vi "Get cif_pluginloader_DiscoverResponse.vi"(8 "error in (no error)":errorcluster, 11 "gRPCid":T1) -> (0 "error out":errorcluster, 2 "package_templatemessage":T2, 3 "gRPCid out":T1)   [LabVIEW 2021, in "CIF_PluginLoader_server.lvlib"]
uses:
  CIF_PluginLoader_server.lvlib
  cif_pluginloader_DiscoverResponse.ctl
  cif_pluginloader_DiscoveredPlugin.ctl
  cif_common_Version.ctl
  cif_management_common_PluginMetadata.ctl
  cif_common_Status.ctl
  <vilib>/gRPC/LabVIEW gRPC Library/Shared/grpcId.ctl
  cif_pluginloader_DiscoverResponse_Flat.ctl
  cif_pluginloader_DiscoveredPlugin_Flat.ctl
  cif_common_Version_Flat.ctl
  cif_management_common_PluginMetadata_Flat.ctl
  cif_common_Status_Flat.ctl
  2ed25e12-861d-4677-8ead-ace2906b2041.vi
  <vilib>/gRPC/LabVIEW gRPC Library/Shared/TranslateGrpcError.vi
  FlatToRichcif_pluginloader_DiscoveredPlugin.vi
  FlatToRichcif_common_Status.vi
  FlatToRichcif_common_Version.vi
  FlatToRichcif_management_common_PluginMetadata.vi
  <vilib>/gRPC/LabVIEW gRPC Library/Server API/Server/Get Server DLL Path.vi
  <vilib>/Utility/error.llb/Error Cluster From Error Code.vi
  <vilib>/gRPC/LabVIEW gRPC Library/grpc-lvsupport-release.lvlib
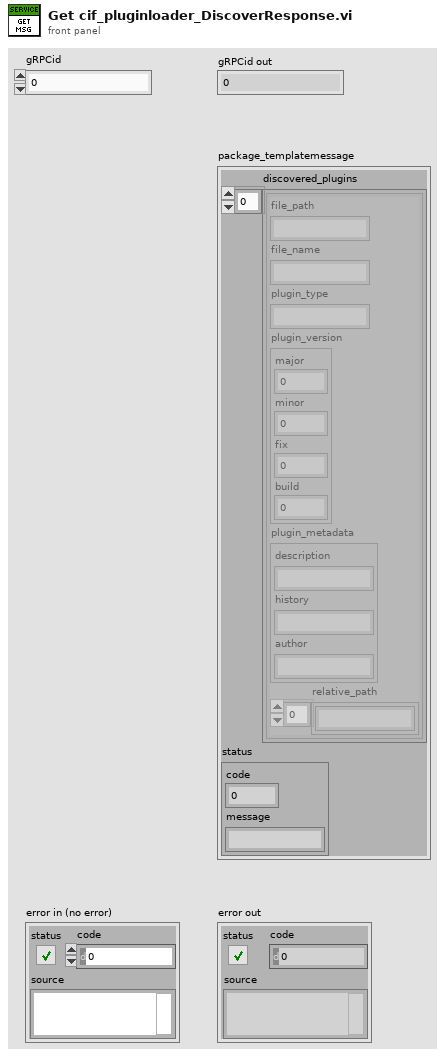
[diagram p1: front panel]
types:
  T1 = typedef "grpc-lvsupport-release.lvlib/grpcId.ctl" = u64
  T2 = typedef "CIF_PluginLoader_server.lvlib/cif_pluginloader_DiscoverResponse.ctl" = cluster{"discovered_plugins":T3[], "status":T6}
  T3 = typedef "CIF_PluginLoader_server.lvlib/cif_pluginloader_DiscoveredPlugin.ctl" = cluster{"file_path":string, "file_name":string, "plugin_type":string, "plugin_version":T4, "plugin_metadata":T5, "relative_path":string[]}
  T4 = typedef "CIF_PluginLoader_server.lvlib/cif_common_Version.ctl" = cluster{"major":u32, "minor":u32, "fix":u32, "build":u32}
  T5 = typedef "CIF_PluginLoader_server.lvlib/cif_management_common_PluginMetadata.ctl" = cluster{"description":string, "history":string, "author":string}
  T6 = typedef "CIF_PluginLoader_server.lvlib/cif_common_Status.ctl" = cluster{"code":i32, "message":string}
  T7 = typedef "CIF_PluginLoader_server.lvlib/cif_pluginloader_DiscoverResponse_Flat.ctl" = cluster{"discovered_plugins":T8[], "status":T11}
  T8 = typedef "CIF_PluginLoader_server.lvlib/cif_pluginloader_DiscoveredPlugin_Flat.ctl" = cluster{"file_path":string, "file_name":string, "plugin_type":string, "plugin_version":T9, "plugin_metadata":T10, "relative_path":string[]}
  T9 = typedef "CIF_PluginLoader_server.lvlib/cif_common_Version_Flat.ctl" = cluster{"major":u32, "minor":u32, "fix":u32, "build":u32}
  T10 = typedef "CIF_PluginLoader_server.lvlib/cif_management_common_PluginMetadata_Flat.ctl" = cluster{"description":string, "history":string, "author":string}
  T11 = typedef "CIF_PluginLoader_server.lvlib/cif_common_Status_Flat.ctl" = cluster{"code":i32, "message":string}
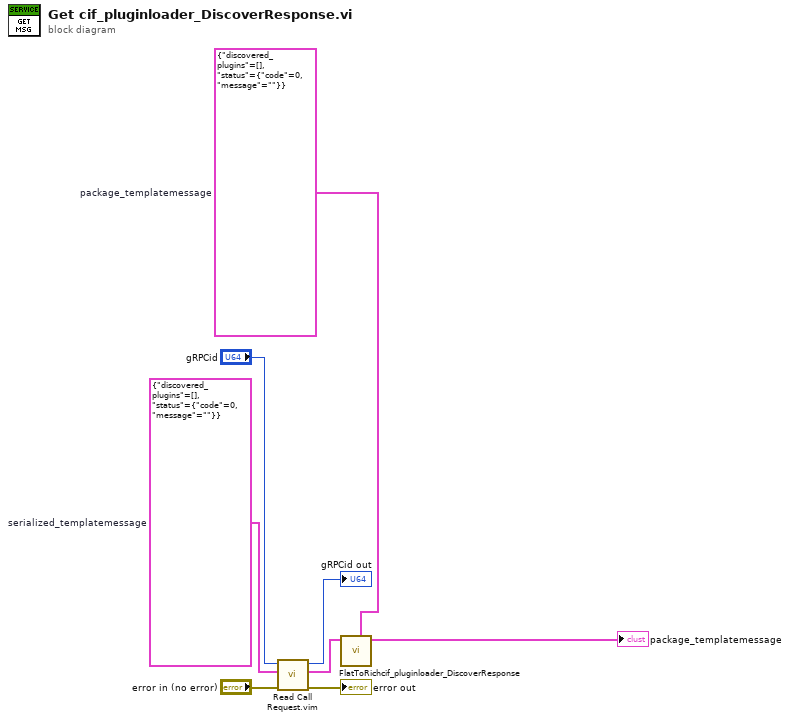
[diagram p0: block diagram]
diagram:
  w6 = T7 {"discovered_plugins"=[], "status"={"code"=0, "message"=""}}  # serialized_templatemessage
  w5 = T2 {"discovered_plugins"=[], "status"={"code"=0, "message"=""}}  # package_templatemessage
  n1 = call "Read Call Request.vim"("error in"="error in (no error)", "Request Type"=w6, "gRPCid in"="gRPCid") -> ("error out"=→"error out":errorcluster, "Request Data"=w4:T7, "gRPCid out"=→"gRPCid out":T1)  [unwired: 6 in]
  n2 = call "FlatToRichcif_pluginloader_DiscoverResponse.vi"("OutputClusterType"=w5, "InputCluster"=w4) -> ("OutputCluster"=→"package_templatemessage":T2)  [unwired: 9 in]
